vi "WBFM_Simulation.vi"() -> ()   [LabVIEW 2013]
uses:
  <vilib>/Analysis/3filter.llb/IIR Filter (DBL).vi
  <vilib>/Analysis/3filter.llb/FIR Filter (DBL).vi
  <vilib>/addons/Modulation/Analog/MT Passband PLL.vi
  <vilib>/express/express analysis/Spectral/Block/exnSpectralBlock spectral measurements RMS poly.vi
  <vilib>/express/express analysis/Spectral/Block/exnSpectralBlock spectral measurements RMS DDT.vi
  <vilib>/express/express analysis/Spectral/XNode/ExpressSpectralMeasurementsBlockNode.xnode
  <vilib>/addons/Modulation/niAMT.lvlib
  <vilib>/Analysis/NI_AALPro.lvlib
  <vilib>/Analysis/NI_AALBase.lvlib
panel:
  out "Estimated Freq.":dbl=100000.0 caption="Frequency"
  in  "Mod. Freq.":dbl=2000.0 caption="Frequency"
  in  "WAV SR":dbl=44100.0 caption="dt"
  in  "LPF Cut-Off":dbl=5000.0 caption="Lower Cut-Off"
  in  "SNR (dB)":dbl(slide)=30.0 caption="Standard deviation" scale=-20.0..50.0
  out "Recovered Signal":dynamicdata(graph)
  out "Baseband":dynamicdata(graph)
  out "FM FFT":dynamicdata(graph)
  out "FM Wave":dynamicdata(graph)
  in  "Carrier Amp.":dbl=1.0 caption="Amplitude"
  in  "stop":bool
  in  "Frequency Deviation":dbl(slide)=200.0 scale=0.0..20000.0
  in  "Carrier Freq.":dbl=100000.0 caption="Frequency"
  # "Frequency Modulation"
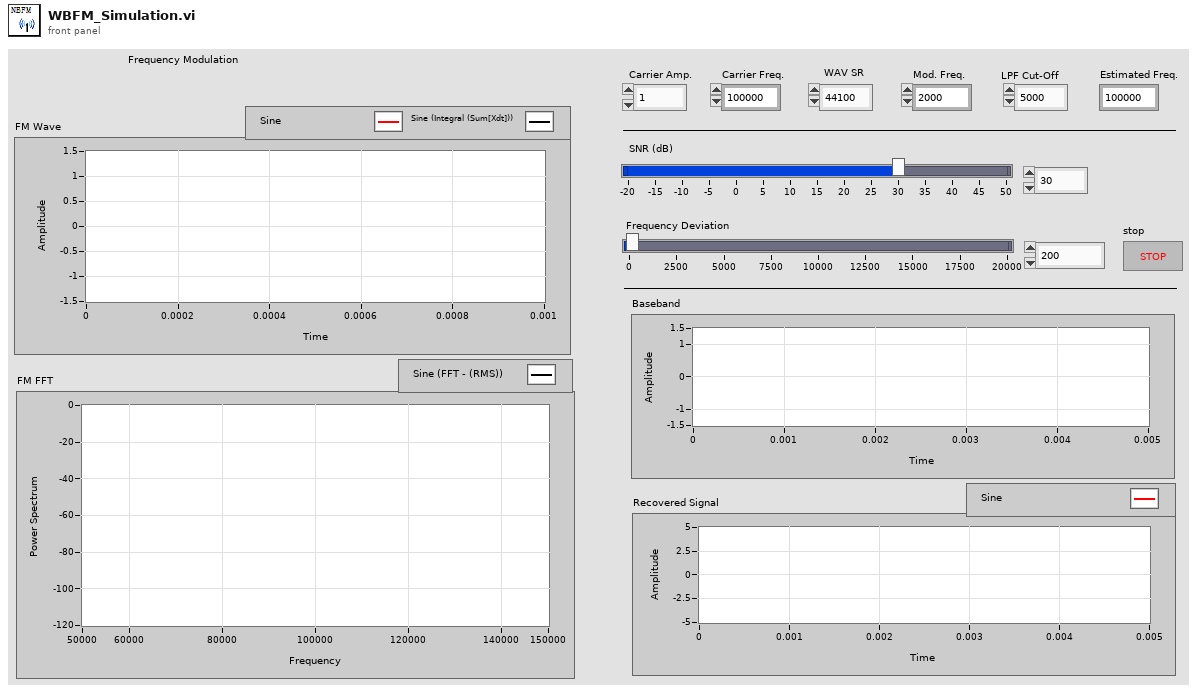
[diagram p1: front panel]
types:
  T1 = cluster{"averaging mode":u16, "weighting mode":u16, "number of averages":u32}
  T2 = cluster{"dB On (F)":bool, "unwrap phase (F)":bool, "convert to degree (F)":bool}
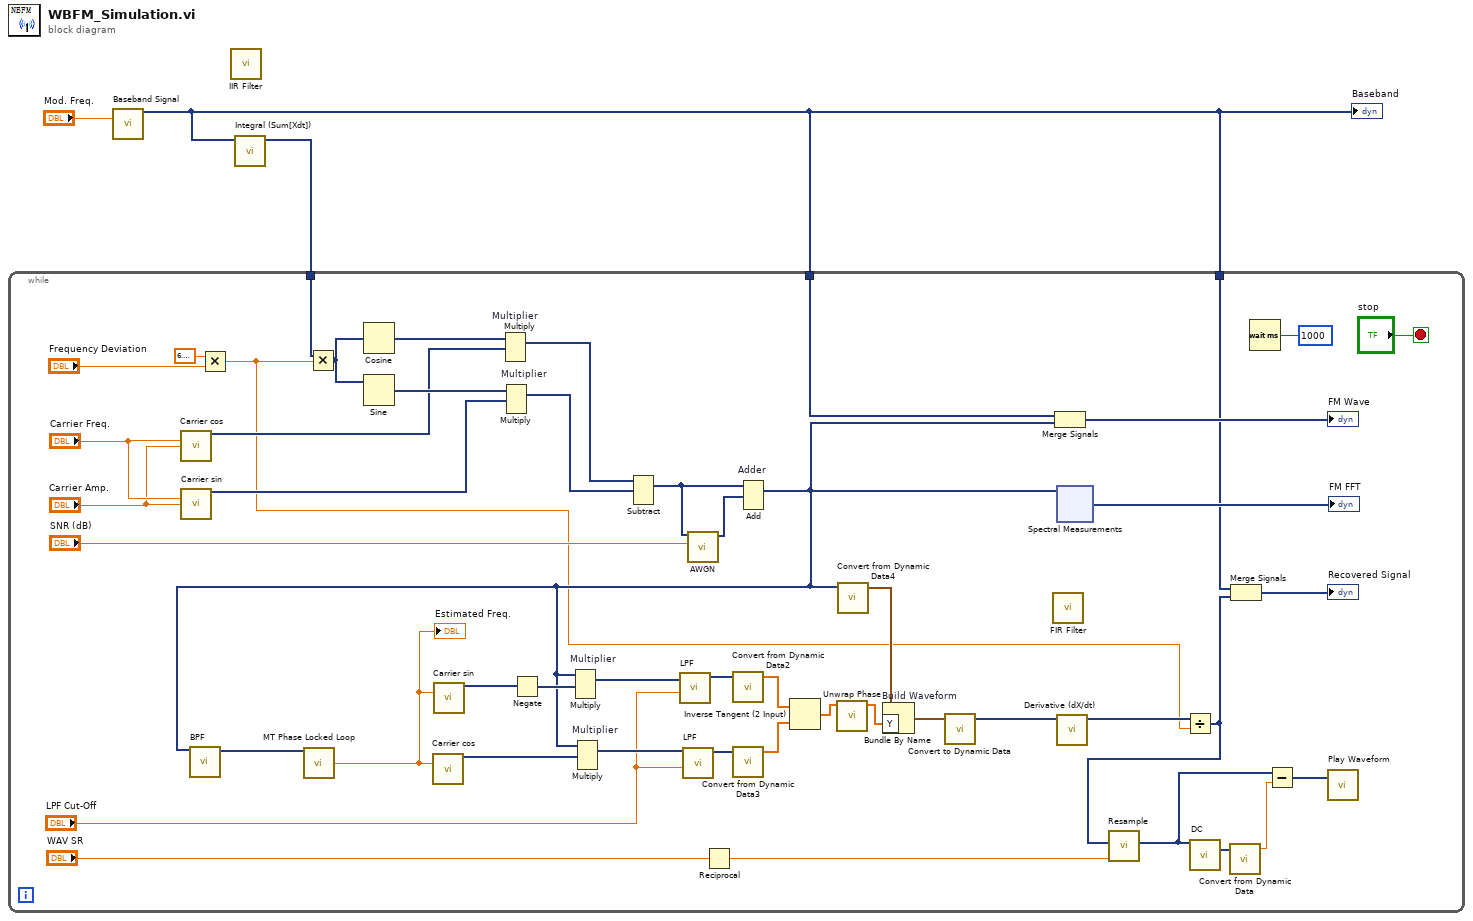
[diagram p0: block diagram]
diagram:
  n1 = call "Baseband Signal"("Frequency"="Mod. Freq.") -> ("Sine"=w1:dynamicdata)  [unwired: 13 in, 1 out]
  "Baseband" <- w1
  n2 = call-poly <vilib>:"IIR Filter.vi"() -> ()  [unwired: 4 in, 2 out]
  n3 = call "Integral (Sum[Xdt])"("Signals"=w1) -> ("Result"=w2:dynamicdata)  [unwired: 5 in, 1 out]
  n4 = while {
    tunnel: w1 -> [w8]
    tunnel: w2 -> [w47]
    tunnel: w1 -> [w5]
    stop <- "stop" stop-if-true
    n5 = call "Carrier cos"("Frequency"="Carrier Freq.", "Amplitude"="Carrier Amp.") -> ("Sine"=w30:dynamicdata)  [unwired: 12 in, 1 out]
    n6 = call "Carrier sin"("Frequency"="Carrier Freq.", "Amplitude"="Carrier Amp.") -> ("Sine"=w29:dynamicdata)  [unwired: 12 in, 1 out]
    n7 = Multiply ("Multiplier")(x=6.283185307179586, y="Frequency Deviation") -> (x*y=w6:dbl)
    n8 = Multiply ("Multiplier")(x=w47, y=w6) -> (x*y=w33:dynamicdata)
    n9 = Cosine(x=w33) -> (cos(x)=w32:dynamicdata)
    n10 = Sine(x=w33) -> (sin(x)=w31:dynamicdata)
    n11 = Multiply "Multiplier"(1:w30, 2:w32) -> (0:w28:dynamicdata)  [unwired: 1 in, 1 out]
    n12 = Multiply "Multiplier"(1:w29, 2:w31) -> (0:w27:dynamicdata)  [unwired: 1 in, 1 out]
    n13 = Subtract(1:w27, 2:w28) -> (0:w34:dynamicdata)  [unwired: 1 in, 1 out]
    n14 = call "AWGN.vi"("AWGN (dB)"="SNR (dB)", "Dynamic Data"=w34) -> ("DC with Gaussian Noise"=w43:dynamicdata)  [unwired: 9 in]
    n15 = Reciprocal(x="WAV SR") -> (1/x=w35:dbl)
    n16 = Add "Adder"(1:w43, 2:w34) -> (0:w13:dynamicdata)  [unwired: 1 in, 1 out]
    n17 = call "BPF"("Signal"=w13) -> ("Filtered Signal"=w41:dynamicdata)  [unwired: 9 in, 1 out]
    n18 = call-poly <vilib>:"MT Phase Locked Loop.vi"("passband waveform"=w41) -> ("estimated carrier frequency (Hz)"=w26:dbl)  [unwired: 10 in, 4 out]
    "Estimated Freq." <- w26
    n19 = call "Carrier cos"("Frequency"=w26) -> ("Sine"=w18:dynamicdata)  [unwired: 13 in, 1 out]
    n20 = call "Carrier sin"("Frequency"=w26) -> ("Sine"=w20:dynamicdata)  [unwired: 13 in, 1 out]
    n21 = Negate(x=w20) -> (-x=w19:dynamicdata)
    n22 = Multiply "Multiplier"(1:w19, 2:w13) -> (0:w25:dynamicdata)  [unwired: 1 in, 1 out]
    n23 = Multiply "Multiplier"(1:w18, 2:w13) -> (0:w24:dynamicdata)  [unwired: 1 in, 1 out]
    n24 = call "LPF"("Lower Cut-Off"="LPF Cut-Off", "Signal"=w25) -> ("Filtered Signal"=w22:dynamicdata)  [unwired: 8 in, 1 out]
    n25 = call "LPF"("Lower Cut-Off"="LPF Cut-Off", "Signal"=w24) -> ("Filtered Signal"=w21:dynamicdata)  [unwired: 8 in, 1 out]
    n26 = call "Convert from Dynamic Data2"("Dynamic Data Type"=w22) -> ("Array"=w17:dbl[])  [unwired: 3 in]
    n27 = call "Convert from Dynamic Data3"("Dynamic Data Type"=w21) -> ("Array"=w16:dbl[])  [unwired: 3 in]
    n28 = Inverse Tangent (2 Input)(1:w16, 2:w17) -> (0:w15:dbl[])
    n29 = call <vilib>:"Unwrap Phase.vi"("Phase"=w15) -> ("Unwrapped Phase"=w14:dbl[])  [unwired: 9 in, 1 out]
    n30 = call "Convert from Dynamic Data4"("Dynamic Data Type"=w13) -> ("Waveform"=w12:waveform(dbl))  [unwired: 3 in]
    n31 = Bundle By Name "Build Waveform"(cluster=w12, "Y"=w14) -> (w11:waveform(dbl))
    n32 = call "Convert to Dynamic Data"("Waveform"=w11) -> ("Dynamic Data Type"=w10:dynamicdata)  [unwired: 3 in]
    n33 = call-poly <vilib>:"FIR Filter.vi"() -> ()  [unwired: 4 in, 2 out]
    n34 = Merge Signals "Merge Signals"(w8, w13) -> (→"FM Wave":dynamicdata)
    n35 = xnode ("Spectral Measurements")("Signals"=w13) -> ("FFT - (RMS)"=→"FM FFT":dynamicdata)  [unwired: 1 in, 2 out]
    n36 = call "Derivative (dX/dt)"("Signals"=w10) -> ("Result"=w7:dynamicdata)  [unwired: 5 in, 1 out]
    n37 = Divide(x=w7, y=w6) -> (x/y=w4:dynamicdata)
    n38 = call "Resample"("dt"=w35, "Signals"=w4) -> ("Resampled Signals"=w40:dynamicdata)  [unwired: 7 in, 2 out]
    n39 = call "DC"("Signals"=w40) -> ("RMS"=w39:dynamicdata)  [unwired: 13 in, 1 out]
    n40 = call "Convert from Dynamic Data"("Dynamic Data Type"=w39) -> ("Scalar"=w38:dbl)  [unwired: 3 in]
    n41 = Merge Signals "Merge Signals"(w5, w4) -> (→"Recovered Signal":dynamicdata)
    n42 = Wait (ms)(milliseconds to wait=u32 1000) -> ()  [unwired: 1 out]
    n43 = Subtract(x=w40, y=w38) -> (x-y=w37:dynamicdata)
    n44 = call "Play Waveform"("Data"=w37) -> ()  [unwired: 18 in, 1 out]
  }
